vi "To XML - Package is not empty - XML contains package.vi"() -> ()   [LabVIEW 2013, in "JUnit XML Tests.lvlib" / "Test Suite.lvlib"]
uses:
  Test Suite.lvlib
  JUnit XML/Test Suite/Test Suite.lvclass/Test Suite.ctl
  JUnit XML/Test Suite/Test Suite.lvclass
  JUnit XML/Test Suite/Write Timestamp.vi
  <vilib>/addons/_JKI Toolkits/Caraya/classes/Assert/Assert Equal Value_Variant.vi
  <vilib>/addons/_JKI Toolkits/Caraya/classes/Test/Test.lvclass
  <vilib>/addons/_JKI Toolkits/Caraya/classes/Assert/Assert.lvclass
panel:
  out "error out":errorcluster
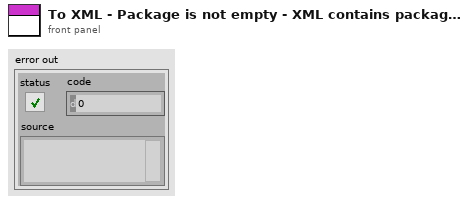
[diagram p1: front panel]
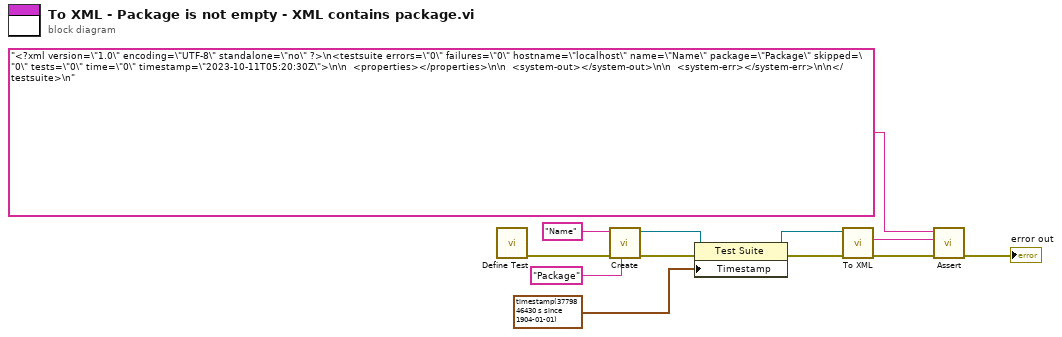
[diagram p0: block diagram]
diagram:
  n1 = call <vilib>:"Define Test.vi"() -> ("error out"=w3:errorcluster)  [unwired: 10 in, 1 out]
  n2 = call "Create.vi"("Package (\"\" = undefined)"="Package" ("Package (\"\" = undefined)"), "error in (no error)"=w3, "Name"="Name" ("Package")) -> ("error out"=w12:errorcluster, "Test Suite"=w8:refnum<class "Test Suite.lvclass">)  [unwired: 7 in]
  n3 = property class="Test Suite"(reference=w8, error in=w12, "Timestamp"=timestamp(3779846430.123 s since 1904-01-01)) -> (reference out=w7:refnum<class "Test Suite.lvclass">, error out=w9:errorcluster)
  n4 = call-dynamic "To XML.vi"("error in (no error)"=w9, "Serializable in"=w7) -> ("error out"=w2:errorcluster, "XML"=w1:string)  [unwired: 8 in]
  n5 = call-poly <vilib>:"Assert.vi"("error in (no error)"=w2, "Actual"=w1, "Expected"="<?xml version=\"1.0\" encoding=\"UTF-8\" standalone=\"no\" ?>\n<testsuite errors=\"0\" failures=\"0\" hostname=\"localhost\" name=\"Name\" package=\"Package\" skipped=\"0\" tests=\"0\" time=\"0\" timestamp=\"2023-10-11T05:20:30Z\">\n\n  <properties></properties>\n\n  <system-out></system-out>\n\n  <system-err></system-err>\n\n</testsuite>\n") -> ("error out"=→"error out":errorcluster)  [unwired: 7 in, 1 out]
